vi "Write Start Polling.vi"(8 "error in (no error)":errorcluster, 10 "Start Polling":bool, 11 "Polling Start Stop Msg in":refnum<class "Polling Start Stop Msg.lvclass">) -> (0 "error out":errorcluster, 3 "Polling Start Stop Msg out":refnum<class "Polling Start Stop Msg.lvclass">)   [LabVIEW 2016, in "CS++BaseActor.lvlib" / "Polling Start Stop Msg.lvclass"]
uses:
  Polling Start Stop Msg.lvclass
  Polling Start Stop Msg.lvclass/Polling Start Stop Msg.ctl
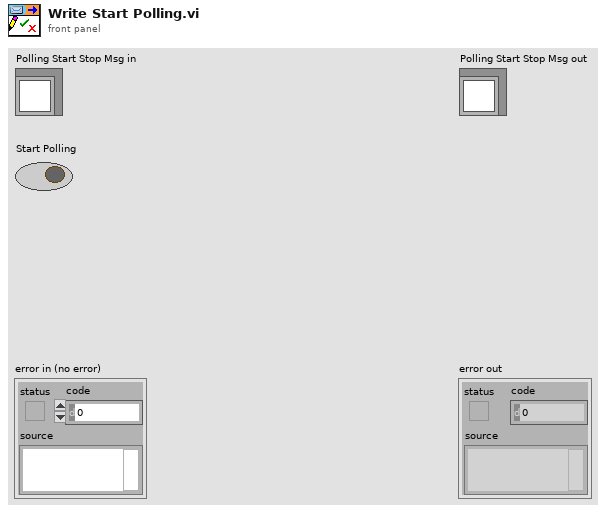
[diagram p1: front panel]
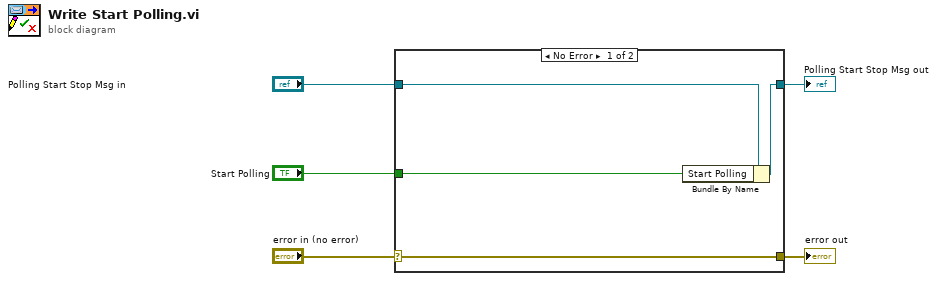
[diagram p0: block diagram]
diagram:
  n1 = case shown="No Error" "error in (no error)" {
    selector: "error in (no error)" -> [w9 w10]
    tunnel: [w9 w10] -> w4
    tunnel: [w7 w11] -> w2
    tunnel: "Polling Start Stop Msg in" -> [w8 w11]
    tunnel: "Start Polling" -> [w6 _]
    frame No Error {
      n2 = Bundle By Name(cluster=w8, "Start Polling"=w6) -> (w7:refnum<class "Polling Start Stop Msg.lvclass">)
    }
    frame Error {
    }
  }
  "error out" <- w4
  "Polling Start Stop Msg out" <- w2
